vi "SMO.UI.Embedded.UIStateChange.vi"(8 "error in (no error)":errorcluster, 10 "UI State":T1=enum."Embedded", 11 "SMO.UI.Embedded":refnum<class "SMO.UI.Embedded.lvclass">) -> (0 "error out":errorcluster, 3 "SMO.UI.Embedded out":refnum<class "SMO.UI.Embedded.lvclass">)   [LabVIEW 2016, in "SMO.UI.Embedded.lvclass"]
doc: "---------------------------------------------------------------\nJKI State Machine Objects™\nhttp://jki.net/state-machine-objects/\nCopyright (C) 2005-2015, JKI <info@jki.net>\nALL RIGHTS RESERVEDJKI State Machine Objects (SMO) 1.0.0.4\nJKI - JKI\nCopyright (c) 2015, JKI"
uses:
  SMO.UI.Embedded.lvclass
  C:/Program Files (x86)/National Instruments/LabVIEW 2016/vi.lib/JKI/JKI SMO/SMO/SMO.lvclass
  Typedefs/UI State.ctl
  Typedefs/PublicEvents--SMO.UI.Embedded.UIStateChange.ctl
  <vilib>/JKI/JKI SMO/SMO/SMO.lvclass
  SMO.UI.Embedded.lvclass/SMO.UI.Embedded.ctl
panel:
  # "For instructions on how to use the JKI State Machine Objects, examples and video tutorials, visit:\nhttp://jki.net/state-machine-objects/\n\nJKI State Machine Objects™\nhttp://jki.net/state-machine-objects/\nCopyright (C) 2005-2015, JKI <info@jki.net>\nALL RIGHTS RESERVED"
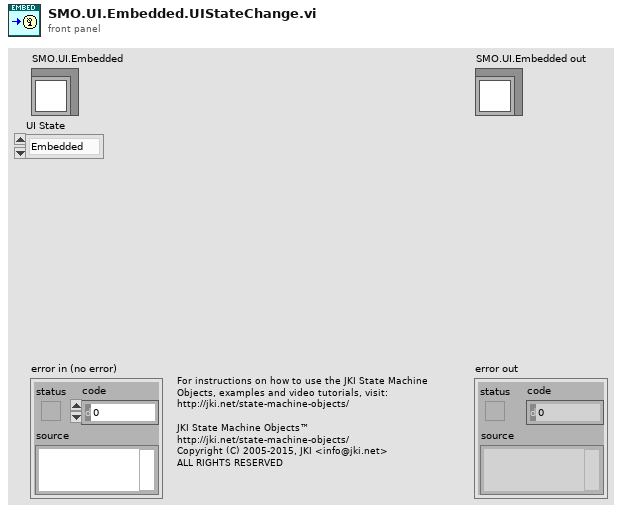
[diagram p1: front panel]
types:
  T1 = typedef "SMO.UI.Embedded.lvclass/UI State.ctl" = enum16{"unknown", "Opened", "Embedded", "Closed"}
  T2 = typedef "SMO.UI.Embedded.lvclass/PublicEvents--SMO.UI.Embedded.UIStateChange.ctl" = cluster{"UI State":T1, "SMO.UI.Embedded":refnum<class "SMO.lvclass">}
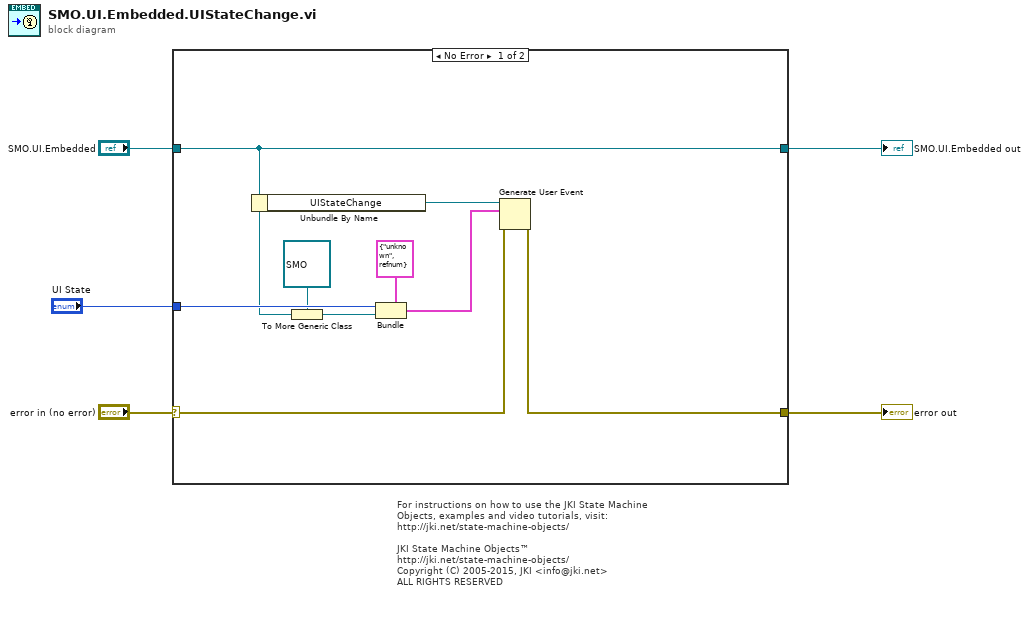
[diagram p0: block diagram]
diagram:
  # "For instructions on how to use the JKI State Machine Objects, examples and video tutorials, visit:\nhttp://jki.net/state-machine-objects/\n\nJKI State Machine Objects™\nhttp://jki.net/state-machine-objects/\nCopyright (C) 2005-2015, JKI <info@jki.net>\nALL RIGHTS RESERVED"
  n1 = case shown="No Error" "error in (no error)" {
    selector: "error in (no error)" -> [w14 w16]
    tunnel: [w12 w16] -> w4
    tunnel: [w8 w15] -> w5
    tunnel: "SMO.UI.Embedded" -> [w8 w15]
    tunnel: "UI State" -> [w11 _]
    frame No Error {
      n2 = Unbundle By Name(w8) -> ("UIStateChange"=w13:refnum<user-event>)
      n3 = To More Generic Class(target class=refnum<class "SMO.lvclass"> refnum ("SMO.UI.Embedded"), reference=w8) -> (generic class reference=w7:refnum<class "SMO.lvclass">)
      n4 = Bundle(cluster=T2 {"UI State"=enum."unknown", "SMO.UI.Embedded"=refnum} ("UI State Change"), "UI State"=w11, "SMO.UI.Embedded"=w7) -> (w10:T2)
      n5 = Generate User Event(user event=w13, event data cluster=w10, error in=w14) -> (error out=w12:errorcluster)  [unwired: 1 in, 1 out]
    }
    frame Error {
    }
  }
  "error out" <- w4
  "SMO.UI.Embedded out" <- w5
